vi "Uses Buffer.vi"(8 "error in (no error)":errorcluster, 11 "DMM6500 in":refnum<class "DMM6500.lvclass">) -> (0 "error out":errorcluster, 2 "Uses Buffer":bool=TRUE, 3 "DMM6500 out":refnum<class "DMM6500.lvclass">)   [LabVIEW 2023, in "HAF.lvlib" / "DMM6500.lvclass"]
doc: "Indicates whether or not this Driver interfaces with an instrument that uses a Buffer to store results (it may be called something different.) This will be used as part of the Command instruction.\n\nThe default is to return False and sub classes should override."
uses:
  DMM6500.lvclass
  DMM6500.lvclass/DMM6500.ctl
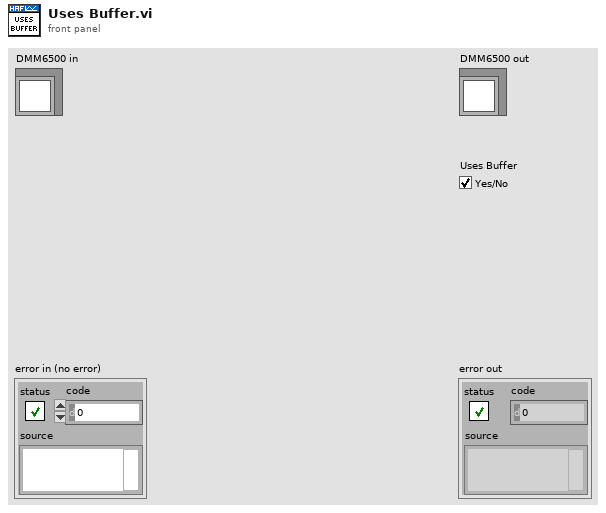
[diagram p1: front panel]
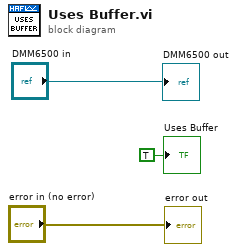
[diagram p0: block diagram]
diagram:
  "error out" <- "error in (no error)"
  "DMM6500 out" <- "DMM6500 in"
  "Uses Buffer" <- TRUE ("Uses Buffer")
